vi "Load config.vi"(8 "error in (no error)":errorcluster) -> (0 "error out":errorcluster, 2 "Mono config":T1={"VISA resource "="", "nm/min"=100.0}, 3 "Lock-in config":T2)   [LabVIEW 2020]
uses:
  controls/Lock-in config.ctl
  controls/Mono config.ctl
  <vilib>/Utility/config.llb/Read Key (String).vi
  <vilib>/Utility/config.llb/Read Key (Double).vi
  <vilib>/Utility/config.llb/NI_LVConfig.lvlib
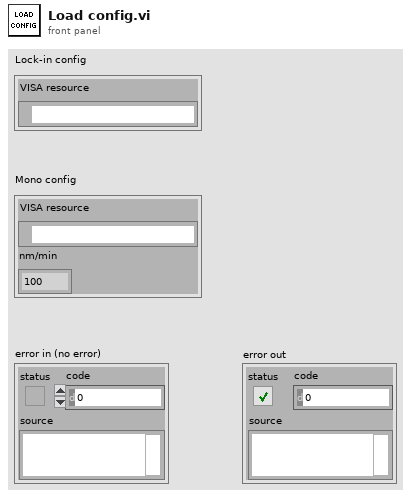
[diagram p1: front panel]
types:
  T1 = typedef "Mono config.ctl" = cluster{"VISA resource ":refnum<visa-resource-name>, "nm/min":dbl}
  T2 = typedef "Lock-in config.ctl" = cluster{"VISA resource ":refnum<visa-resource-name>}
  T3 = typedef "NI_LVConfig.lvlib/Config Data RefNum.ctl" = refnum<k1>
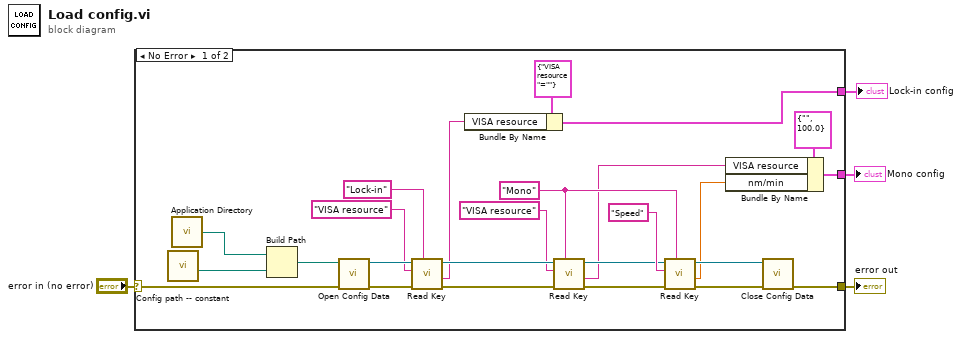
[diagram p0: block diagram]
diagram:
  n1 = case shown="No Error" "error in (no error)" {
    selector: "error in (no error)" -> [w27 w30]
    tunnel: [w26 w30] -> w3
    tunnel: [w7 _] -> w2
    tunnel: [w6 _] -> w1
    frame No Error {
      w17 = "Mono" ("section")
      n2 = call "Config path -- constant.vi"() -> ("name or relative path"=w5:path)  [unwired: 11 in]
      n3 = call <vilib>:"Application Directory.vi"() -> ("Application Directory"=w29:path)
      n4 = Build Path(base path=w29, name or relative path=w5) -> (appended path=w28:path)
      n5 = call <vilib>:"Open Config Data.vi"("error in (no error)"=w27, "configuration file path"=w28) -> ("error out"=w24:errorcluster, "refnum"=w23:T3)  [unwired: 7 in, 1 out]
      n6 = call-poly <vilib>:"Read Key.vi"("section"="Lock-in", "error in (no error)"=w24, "key"="VISA resource", "refnum"=w23) -> ("error out"=w21:errorcluster, "value"=w11:string, "refnum out"=w20:T3)  [unwired: 4 in, 1 out]
      n7 = Bundle By Name(cluster=T2 {"VISA resource "=""} ("Lock-in config"), "VISA resource"=w11) -> (w6:T2)
      n8 = call-poly <vilib>:"Read Key.vi"("section"=w17, "error in (no error)"=w21, "key"="VISA resource", "refnum"=w20) -> ("error out"=w18:errorcluster, "value"=w9:string, "refnum out"=w15:T3)  [unwired: 4 in, 1 out]
      n9 = call-poly <vilib>:"Read Key.vi"("section"=w17, "error in (no error)"=w18, "key"="Speed", "refnum"=w15) -> ("error out"=w14:errorcluster, "value"=w8:dbl, "refnum out"=w13:T3)  [unwired: 4 in, 1 out]
      n10 = Bundle By Name(cluster=T1 {"VISA resource "="", "nm/min"=100.0} ("Mono config"), "VISA resource"=w9, "nm/min"=w8) -> (w7:T1)
      n11 = call <vilib>:"Close Config Data.vi"("error in (no error)"=w14, "refnum"=w13) -> ("error out"=w26:errorcluster)  [unwired: 8 in, 1 out]
    }
    frame Error {
    }
  }
  "Lock-in config" <- w1
  "Mono config" <- w2
  "error out" <- w3
